vi "BlankArray.vi"() -> (3 "Array":bool[](array[boolean]))   [LabVIEW 2020]
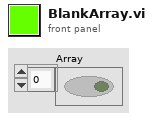
[diagram p1: front panel]
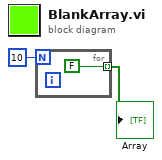
[diagram p0: block diagram]
diagram:
  n1 = for {
    N: 10 -> [_]
    tunnel: [FALSE ("SettingsB")] -> w1 mode=indexing
  }
  "Array" <- w1
